vi "Autozero.vi"(8 "error in (no error)":errorcluster, 10 "Autozero (True)":bool=TRUE, 11 "VISA resource name":refnum<visa-resource-name>) -> (0 "error out":errorcluster, 3 "VISA resource name out":refnum<visa-resource-name>)   [LabVIEW 2023, in "Fluke Molbox 1 Plus.lvlib"]
doc: "Enables the reference pressure transducer AutoZ function. Sets the AutoZ status for both of the the internal RPTs."
uses:
  Fluke Molbox 1 Plus.lvlib
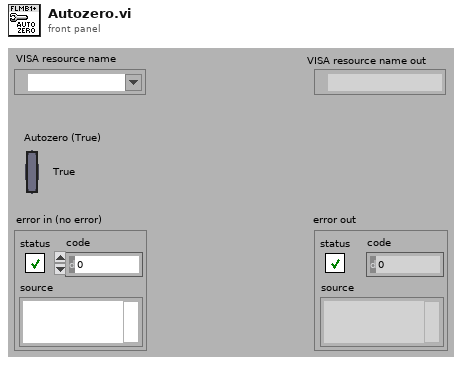
[diagram p1: front panel]
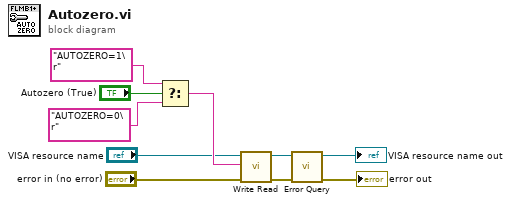
[diagram p0: block diagram]
diagram:
  n1 = Select(t="AUTOZERO=1\r", s="Autozero (True)", f="AUTOZERO=0\r") -> (s? t:f=w6:string)
  n2 = call "Write Read.vi"("error in (no error)"="error in (no error)", "Write String"=w6, "VISA resource name"="VISA resource name") -> ("error out"=w3:errorcluster, "VISA resource name out"=w4:refnum<visa-resource-name>)  [unwired: 6 in, 1 out]
  n3 = call "Error Query.vi"("error in (no error)"=w3, "VISA resource name"=w4) -> ("error out"=→"error out":errorcluster, "VISA resource name out"=→"VISA resource name out":refnum<visa-resource-name>)  [unwired: 6 in, 2 out]
